vi "while con boton de parada.vi"() -> ()   [LabVIEW 2020]
panel:
  in  "milliseconds to wait":u32
  out "millisecond timer value":u32
  in  "stop":bool
  out "floor(x): largest int <= x":dbl
  out "Numeric":i32
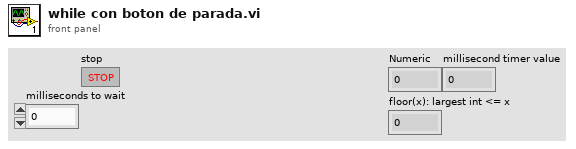
[diagram p1: front panel]
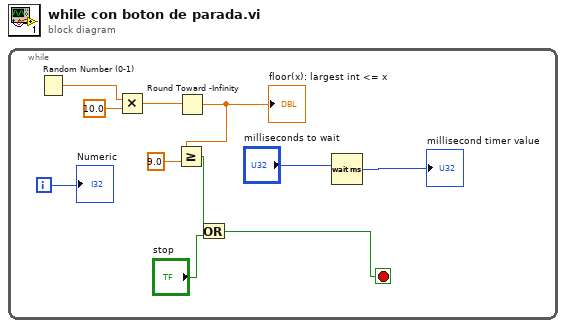
[diagram p0: block diagram]
diagram:
  n1 = while {
    i -> [w4]
    stop <- w2 stop-if-true
    n2 = Random Number (0-1)() -> (number: 0 to 1=w11:dbl)
    n3 = Multiply(x=w11, y=10.0) -> (x*y=w9:dbl)
    n4 = Round Toward -Infinity(1:w9) -> (0:w7:dbl)
    "floor(x): largest int <= x" <- w7
    n5 = Greater Or Equal?(x=w7, y=9.0) -> (x >= y?=w6:bool)
    n6 = Or(x=w6, y="stop") -> (x .or. y?=w2:bool)
    n7 = Wait (ms)(milliseconds to wait="milliseconds to wait") -> (millisecond timer value=→"millisecond timer value":u32)
    "Numeric" <- w4
  }
